vi "Build.vi"() -> ()   [LabVIEW 2010]
doc: "This VI is an example of a VI that can build a VIPM Package when the Build button is pushed or when called from the command line."
uses:
  <vilib>/Utility/error.llb/DialogType.ctl
  Types/Command Line Args.ctl
  Types/Task Info.ctl
  Types/Job Type.ctl
  <userlib>/_OpenG.lib/file/file.llb/File Exists - Scalar__ogtk.vi
  <userlib>/_OpenG.lib/file/file.llb/Valid Path - Traditional__ogtk.vi
panel:
  out "Tests Pass":bool
  out "Unit Test Results":string
  in  "Autobuild Spec":path
  in  "button_build":bool
  out "Progress status":string
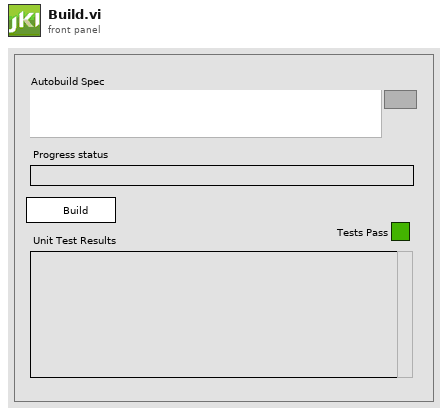
[diagram p1: front panel]
types:
  T1 = enum16{"open", "replace", "create", "open or create", "replace or create", "replace or create with confirmation"}
  T2 = enum32{"invalid app kind", "Development System", "Run Time System", "Student Edition", "Embedded LabVIEW", "Evaluation", "Custom"}
  T3 = typedef "Command Line Args.ctl" = cluster{"BuildNumber":u32, "Error":path, "Running":path, "Workspace":path, "Job":string, "MClog":path, "BuildLog":path, "Copy Built":bool, "SourceVer":string, "MaxBuildVer":string}
  T4 = enum8{"Enabled", "Disabled", "Disabled and Grayed Out"}
  T5 = enum32{"Invalid", "Standard", "Closed", "Hidden", "Minimized", "Maximized"}
  T6 = typedef "Task Info.ctl" = cluster{"Build Spec":string, "Path":path, "Target":string, "Type":T7, "Raw Command":string}
  T7 = typedef "Job Type.ctl" = enum16{"MC", "NOP", "VI", "Build", "VIP", "VIPB", "VIA"}
  T8 = cluster{"Core":cluster{"Current VI Reference":refnum<vi>, "Close Panel on Exit?":bool}, "Build":cluster{"Unit Test":path, "Builds":T6[], "Retain Build":bool}, "Building":bool, "RunningAsCmdLine":bool, "CmdLineArgs":T3, "Autobuild Spec":path, "MCSpec":path}
  T9 = typedef "DialogType.ctl" = u16
  T10 = cluster{"Unit Test":path, "Builds":T6[], "Retain Build":bool}
  T11 = cluster{"Current VI Reference":refnum<vi>, "Close Panel on Exit?":bool}
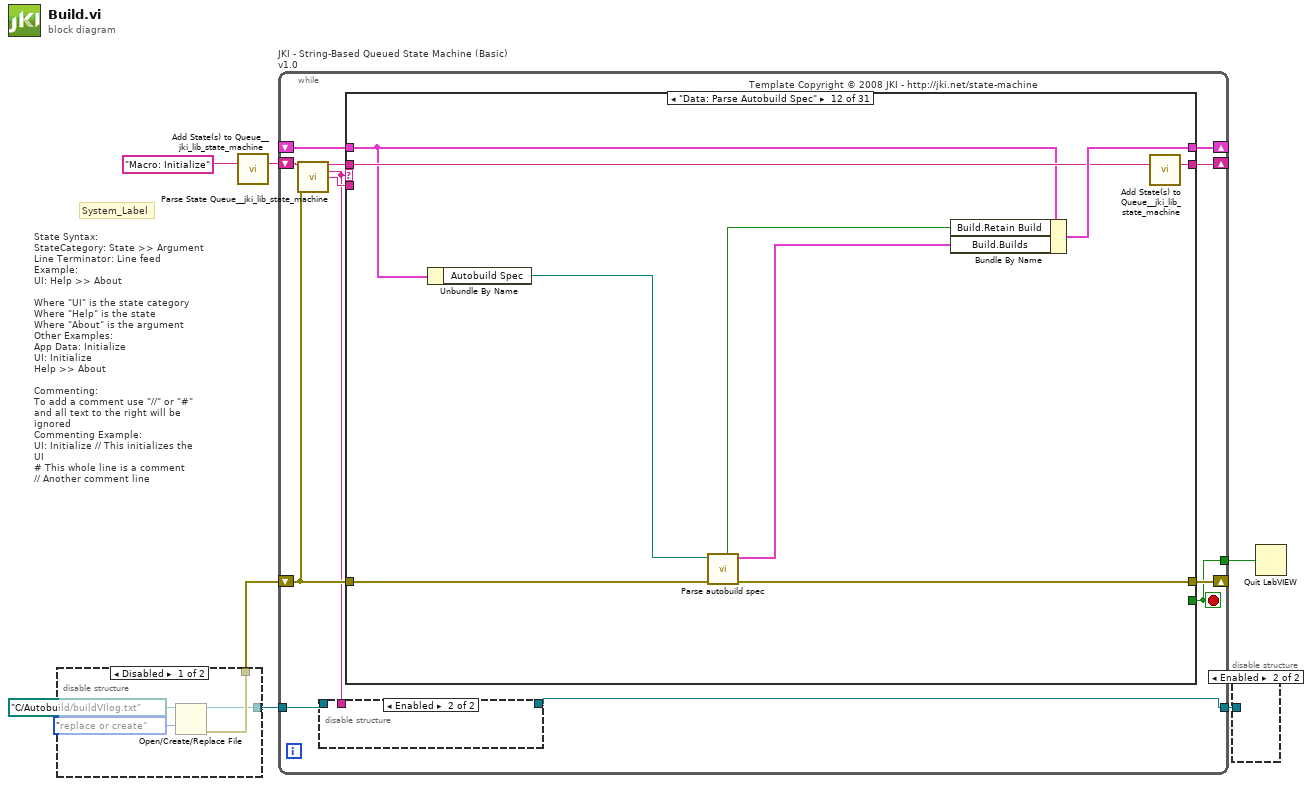
[diagram p0: block diagram]
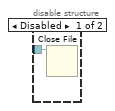
[diagram p2: hidden frame]
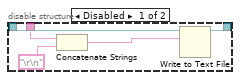
[diagram p4: hidden frame]
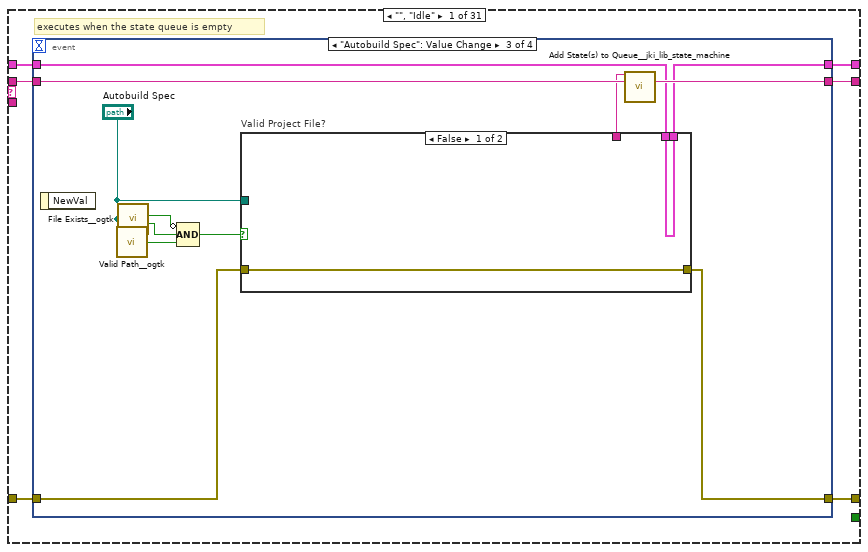
[diagram p5: hidden frame]
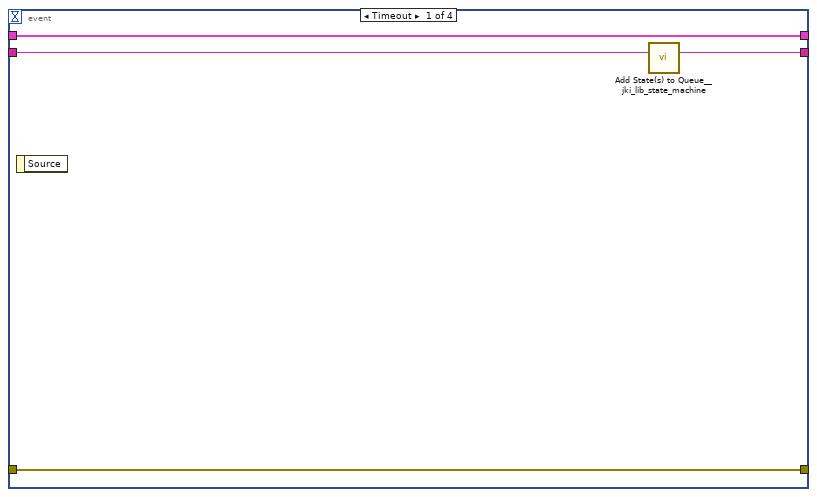
[diagram p6: hidden frame]
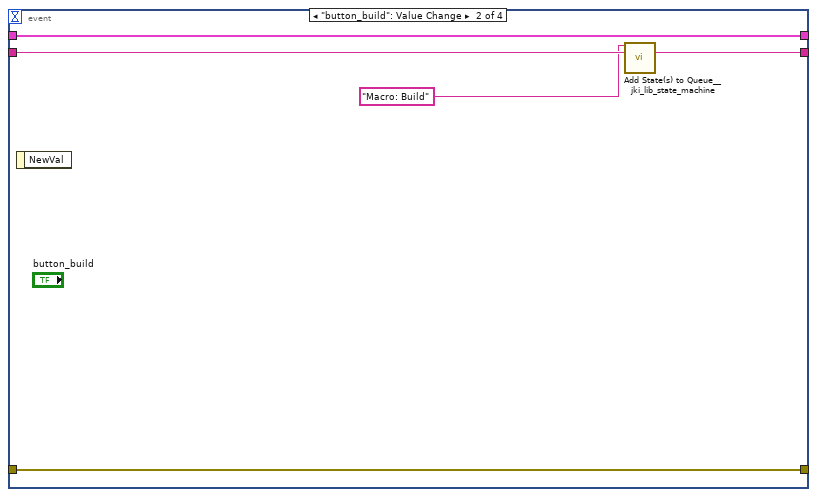
[diagram p7: hidden frame]
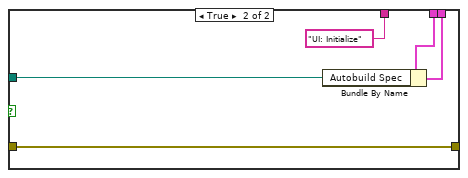
[diagram p8: hidden frame]
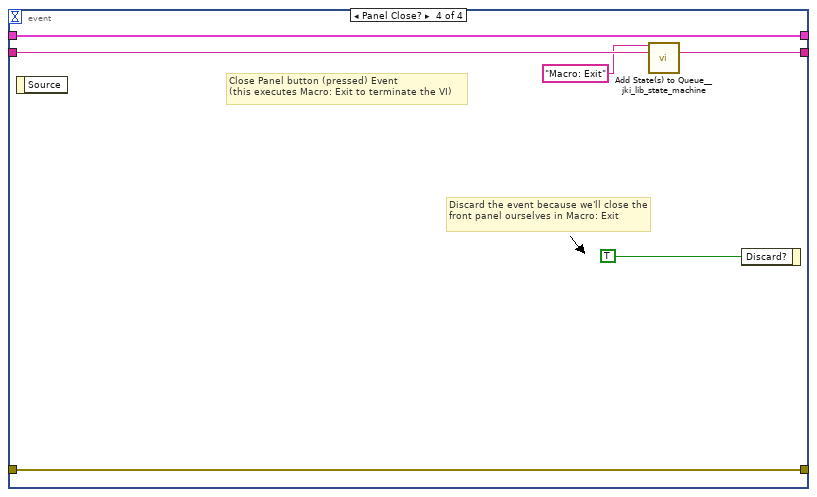
[diagram p9: hidden frame]
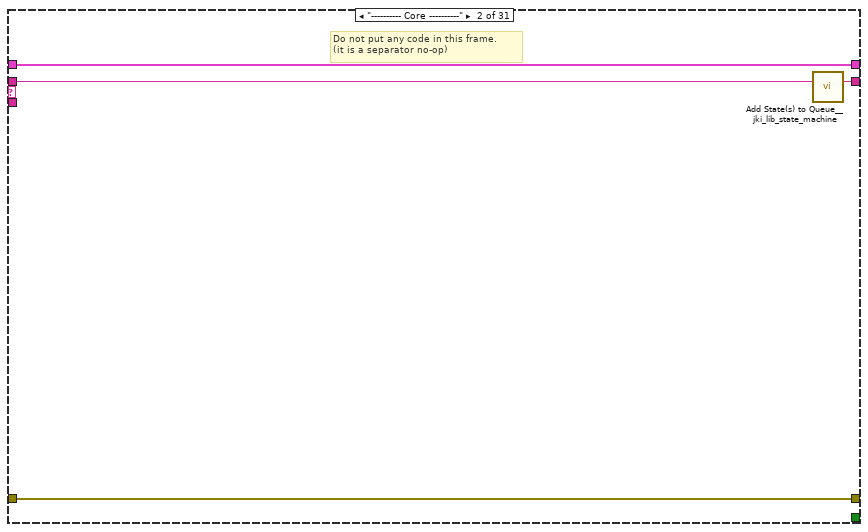
[diagram p10: hidden frame]
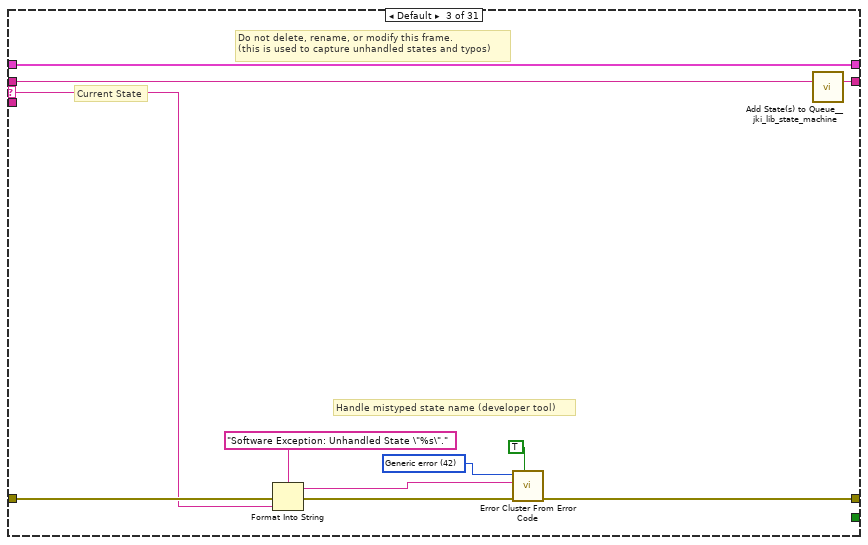
[diagram p11: hidden frame]
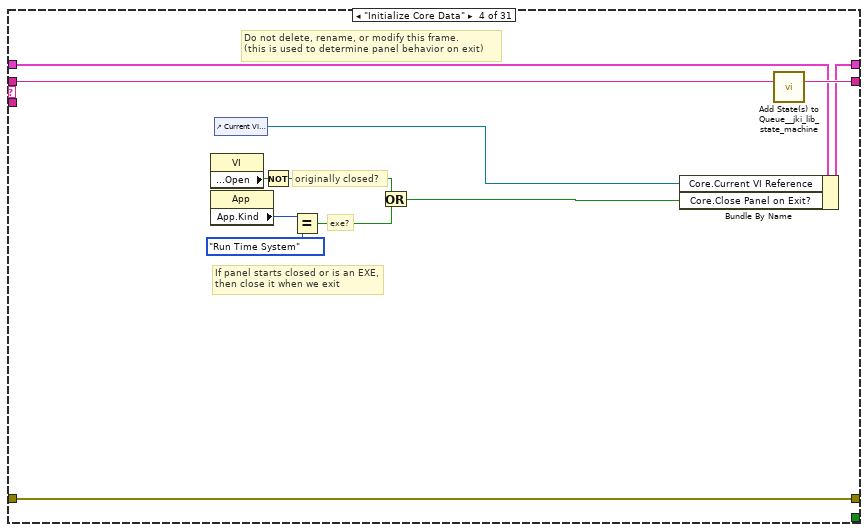
[diagram p12: hidden frame]
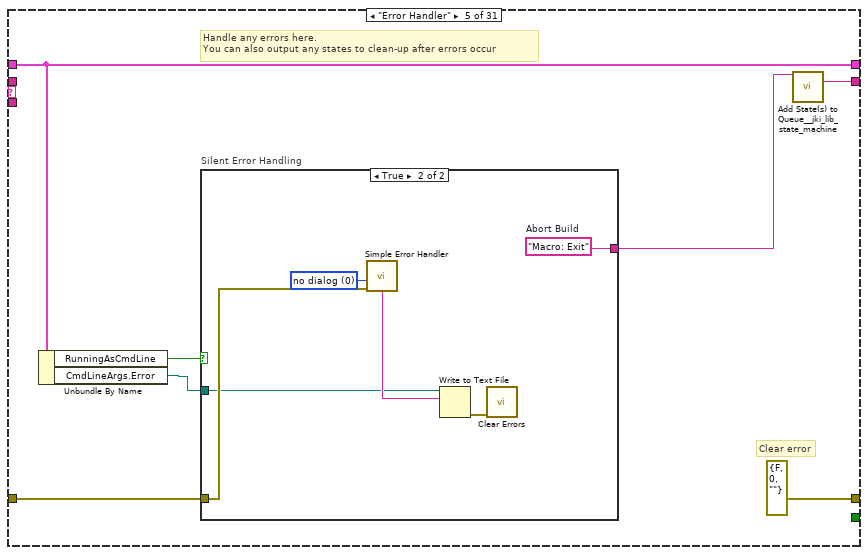
[diagram p13: hidden frame]
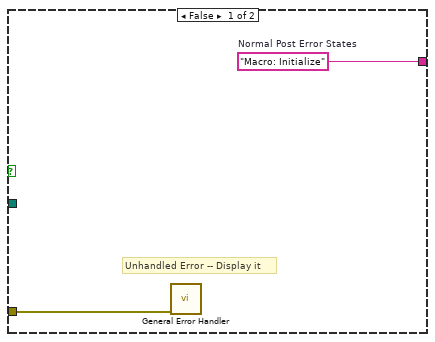
[diagram p14: hidden frame]
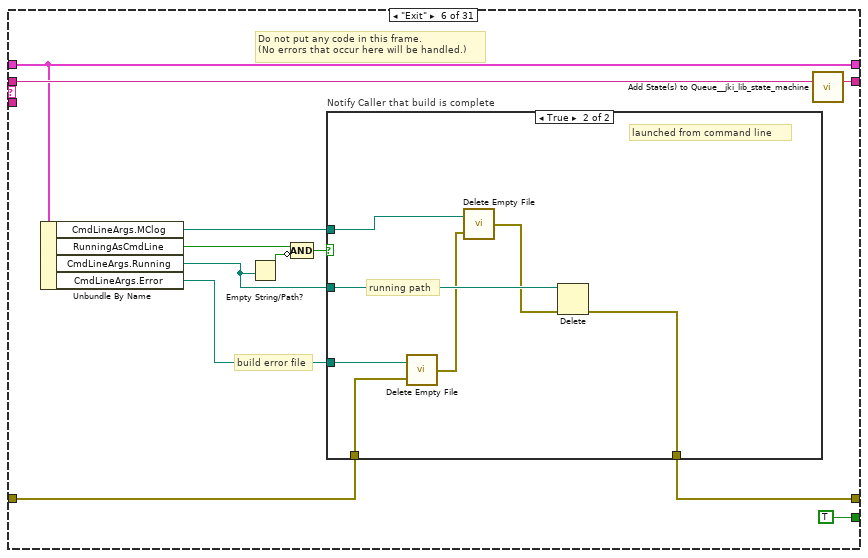
[diagram p15: hidden frame]
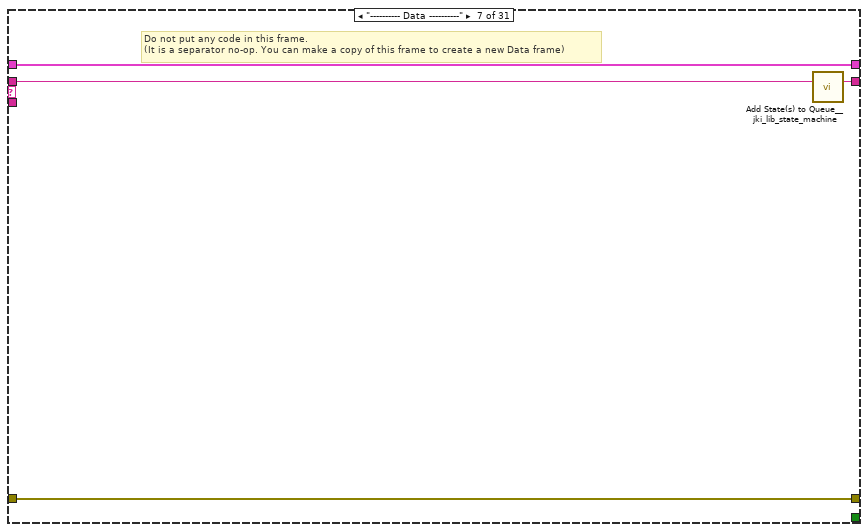
[diagram p17: hidden frame]
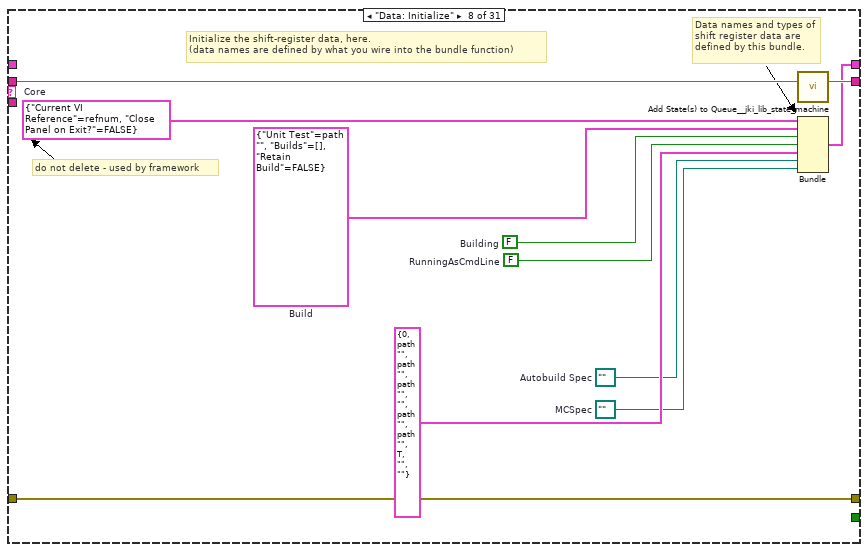
[diagram p18: hidden frame]
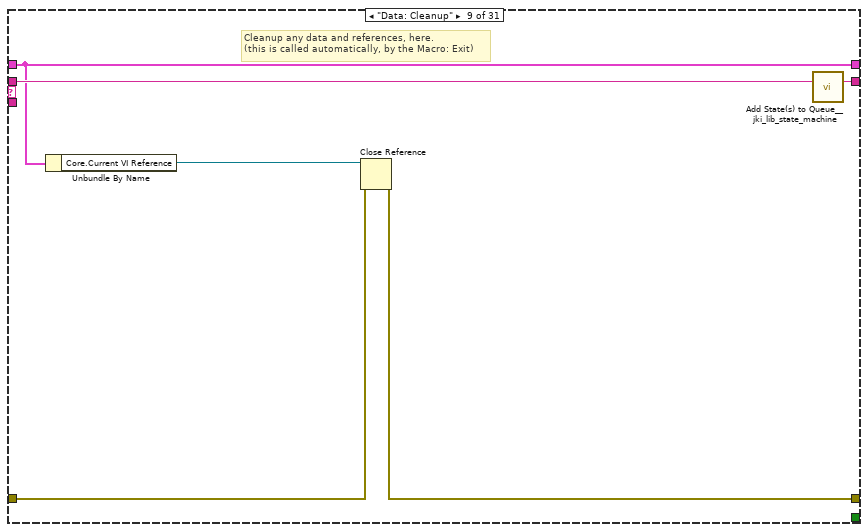
[diagram p19: hidden frame]
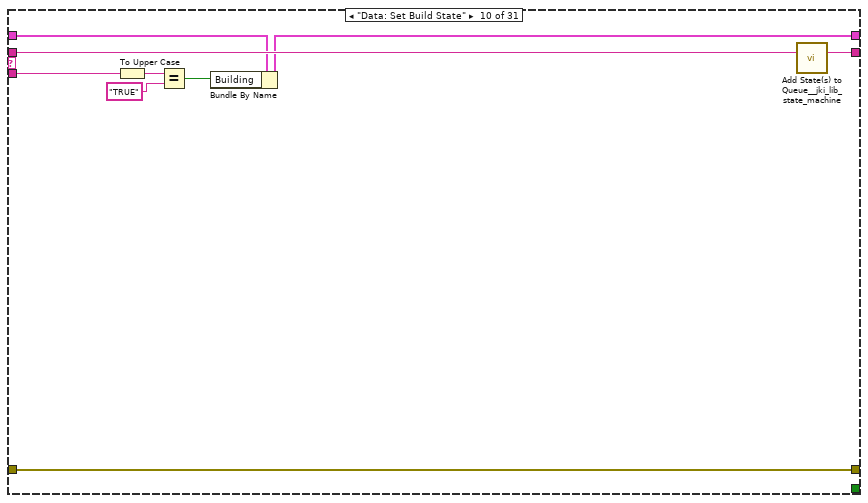
[diagram p20: hidden frame]
diagram:
  # "State Syntax:\nStateCategory: State >> Argument\nLine Terminator: Line feed\nExample:\nUI: Help >> About\n\nWhere \"UI\" is the state category\nWhere \"Help\" is the state\nWhere \"About\" is the argument\nOther Examples:\nApp Data: Initialize\nUI: Initialize\nHelp >> About\n\nCommenting:\nTo add a comment use \"//\" or \"#\" and all text to the right will be ignored\nCommenting Example:\nUI: Initialize // This initializes the UI\n# This whole line is a comment\n// Another comment line"
  # "System_Label"
  n1 = disable-structure shown="Disabled" {
    disable-tunnel: [w10 _] -> w4
    disable-tunnel: [w8 _] -> w3
    frame Disabled {
      n2 = Open/Create/Replace File(file path (use dialog)=path "C:/Autobuild/buildVIlog.txt", operation (0:open)=T1."replace or create") -> (refnum out=w8:refnum<file>, error out=w10:errorcluster)  [unwired: 4 in, 1 out]
    }
    frame Enabled {
    }
  }
  n3 = call <vilib>:"Add State(s) to Queue__jki_lib_state_machine.vi"("State(s) in (\"\")"="Macro: Initialize") -> ("States Out"=w5:string)  [unwired: 14 in]
  n4 = while "JKI - String-Based Queued State Machine (Basic) v1.0" {
    shift-right: [w17] -> _
    shift-left: _ -> [w16]
    shift-right: [w19] -> _
    shift-left: w4 -> [w15]
    shift-right: [w18] -> _
    shift-left: w5 -> [w20]
    tunnel: w3 -> [w14]
    tunnel: [w11] -> w2
    tunnel: [w12] -> w1
    stop <- w12 stop-if-true
    # "Template Copyright © 2008 JKI - http://jki.net/state-machine"
    n5 = call <vilib>:"Parse State Queue__jki_lib_state_machine.vi"("State Queue"=w20, "Error In (no error)"=w15) -> ("Remaining States"=w22:string, "Current State"=w13:string, "Arguments"=w21:string)  [unwired: 11 in]
    n6 = disable-structure shown="Enabled" {
      disable-tunnel: w14 -> [w27 _]
      disable-tunnel: w13 -> [w26 _]
      disable-tunnel: [w23 _] -> w11
      frame Disabled {
        n7 = Concatenate Strings(w26, "\r\n") -> (w25:string)
        n8 = Write to Text File(file (use dialog)=w27, text=w25) -> (refnum out=w23:refnum<file>)  [unwired: 2 in, 2 out]
      }
      frame Enabled {
      }
    }
    n9 = case shown="\"Data: Parse Autobuild Spec\"" w13 {
      selector: w13 -> [_ _ w72 _ _ _ _ _ _ _ _ _ _ _ _ _ _ _ _ _ _ _ _ _ _ _ _ _ _ _ _]
      tunnel: w22 -> [w33 w71 w76 w94 _ w121 w133 w144 w150 w159 w198 w207 w213 w222 w227 w232 w240 w246 w257 w283 w288 w293 w298 w303 w313 w317 w336 w359 w382 w406 w421]
      tunnel: w21 -> [_ _ _ _ _ _ _ _ _ w153 _ _ _ _ _ w228 _ w241 w251 _ _ _ _ _ _ _ _ _ _ _ _]
      tunnel: w16 -> [w31 w68 w74 w85 w99 w111 w130 _ w145 w157 w196 w206 w210 w220 w225 w230 w238 w244 w253 w280 w285 w290 w296 w300 w310 w314 w338 w357 w380 w404 w419]
      tunnel: [w30 w69 w78 w91 errorcluster {"status"=FALSE, "code"=0, "source"=""} ("error out") w110 w131 w140 w146 w156 w192 w202 w211 w216 w224 w229 w237 w242 w254 w281 w286 w291 w295 w301 w311 w315 w324 w354 w372 w401 w413] -> w19
      tunnel: w15 -> [w29 w69 w77 w91 w97 w118 w131 w140 w147 w156 w192 w205 w211 w219 w224 w229 w237 w243 w255 w281 w286 w291 w295 w301 w311 w315 w329 w356 w379 w403 w416]
      tunnel: [w32 w70 w75 w93 w101 w120 w132 w143 w149 w158 w197 w209 w212 w221 w226 w231 w239 w245 w256 w282 w287 w292 w297 w302 w312 w316 w339 w358 w381 w405 w420] -> w18
      tunnel: [_ _ _ _ _ TRUE _ _ _ _ _ _ _ _ _ _ _ _ _ _ _ _ _ _ _ _ _ _ _ _ _] -> w12
      tunnel: [w28 w68 w74 w92 w99 w111 w130 w142 w145 w155 w195 w208 w210 w220 w225 w230 w238 w244 w253 w280 w285 w290 w296 w300 w310 w314 w338 w357 w380 w404 w419] -> w17
      frame "", "Idle" {
        # "executes when the state queue is empty"
        n10 = event shown="[2] \"Autobuild Spec\": Value Change" {
          selector: _ -> [_ _ _ _]
          dyn-events: _ -> [_ _ _ _]
          timeout: _ -> [_ _ _ _]
          tunnel: w33 -> [w37 w42 w54 w67]
          tunnel: [w36 w41 w53 w66] -> w32
          tunnel: w31 -> [w34 w38 w48 w64]
          tunnel: [w35 w39 w44 w65] -> w30
          tunnel: w29 -> [w35 w39 w45 w65]
          tunnel: [w34 w38 w47 w64] -> w28
          event Timeout {
            n11 = event-data() -> ()  [unwired: 1 in, 1 out]
            n12 = call <vilib>:"Add State(s) to Queue__jki_lib_state_machine.vi"("State(s) in (\"\")"=w37) -> ("States Out"=w36:string)  [unwired: 14 in]
          }
          event "button_build": Value Change {
            n13 = event-data() -> ()  [unwired: 1 in, 1 out]
            n14 = call <vilib>:"Add State(s) to Queue__jki_lib_state_machine.vi"("State(s) in Front (\"\")"="Macro: Build", "State(s) in (\"\")"=w42) -> ("States Out"=w41:string)  [unwired: 13 in]
          }
          event "Autobuild Spec": Value Change {
            n15 = event-data() -> ()  [unwired: 1 in, 1 out]
            n16 = call-poly <userlib>:"Valid Path__ogtk.vi"("path"="Autobuild Spec") -> ("valid"=w52:bool)
            n17 = call-poly <userlib>:"File Exists__ogtk.vi"("file path"="Autobuild Spec") -> ("is directory"=w50:bool, "exists"=w51:bool)  [unwired: 6 in]
            n18 = Compound Arithmetic op=AND(invert w50, w51, w52) -> (w49:bool)
            n19 = case "Valid Project File?" shown="False" w49 {
              tunnel: w45 -> [w56 w57]
              tunnel: "Autobuild Spec" -> [_ w59]
              tunnel: w48 -> [w55 w61]
              tunnel: [w55 w60] -> w47
              tunnel: [_ "UI: Initialize"] -> w46
              tunnel: [w56 w57] -> w44
              frame False {
              }
              frame True {
                n20 = Bundle By Name(cluster=w61, "Autobuild Spec"=w59) -> (w60:T8)
              }
            }
            n21 = call <vilib>:"Add State(s) to Queue__jki_lib_state_machine.vi"("State(s) in Front (\"\")"=w46, "State(s) in (\"\")"=w54) -> ("States Out"=w53:string)  [unwired: 13 in]
          }
          event Panel Close? {
            # "Discard the event because we'll close the front panel ourselves in Macro: Exit"
            # "Close Panel button (pressed) Event\n(this executes Macro: Exit to terminate the VI)"
            n22 = event-data() -> ()  [unwired: 1 in, 1 out]
            n23 = call <vilib>:"Add State(s) to Queue__jki_lib_state_machine.vi"("State(s) in Front (\"\")"="Macro: Exit", "State(s) in (\"\")"=w67) -> ("States Out"=w66:string)  [unwired: 13 in]
            n24 = event-data("Discard?"=TRUE) -> ()  [unwired: 1 in, 1 out]
          }
        }
      }
      frame "---------- Core ----------" {
        # "Do not put any code in this frame.\n(it is a separator no-op)"
        n25 = call <vilib>:"Add State(s) to Queue__jki_lib_state_machine.vi"("State(s) in (\"\")"=w71) -> ("States Out"=w70:string)  [unwired: 14 in]
      }
      frame Default {
        w81 = 42 items=["No error", "Argument error", "Memory is full", "Out of zone", "End of file", "File already open", "Generic file I/O error", "File not found", "File permission error", "Disk is full", "Duplicate path", "Too many files open", "System feature not enabled", "Resource file not found", "Cannot add resource", "Resource not found", "Image not found", "Image memory error", "Pen does not exist", "Config type invalid", "Config token not found", "Config parse error", "Config memory error", "Bad external code format", "Bad external code offset", "External code not present", "Null window", "Destroy window error", "Null menu", "Print aborted", "Bad print record", "Print driver error", "Windows error during printing", "Memory error during printing", "Print dialog error", "Generic print error", "Invalid device refnum", "Device not found", "Device parameter error", "Device unit error", "Cannot open device", "Device call aborted", "Generic error", "Cancelled by user", "Object ID too low", "Object ID too high", "Object not in heap", "Unknown heap", "Unknown object (invalid DefProc)", "Unknown object (DefProc not in table)", "Message out of range", "Invalid (null) method", "Unknown message", "Manager call not supported", "Bad address", "Network operation in progress", "Network operation timed out", "Connection is busy", "Network attribute not supported", "Network error", "Address in use", "System out of memory", "Connection aborted", "Connection refused", "Not connected", "Already connected", "Connection closed", "Initialization error (interapplication manager)", "Bad occurrence", "Wait on unbound occurrence handler", "Occurrence queue overflow", "Datalog type conflict", "Unused", "Unrecognized type (interapplication manager)", "Memory corrupt", "Failed to make temporary DLL", "Old CIN version", "Drag socket not found", "Failed to load drop-object", "Failed to register OLE object", "Failed to release OLE object", "Format specifier type mismatch", "Unknown format specifier", "Too few format specifiers", "Too many format specifiers", "Scan failed", "Newer CIN version", "Error converting to variant", "Runtime menu error", "Password tampered", "Variant attribute not found", "Incompatible variant data type", "Event data is not available", "Event Store is not present", "Occurrence is not found", "Event Queue is not created", "Event info is not available", "Refnum passed is NULL", "Error retrieving Class GUID", "Error retrieving CoClass GUID", "Error retrieving TypeLib GUID.", "Bad built application magic bytes.", "Specific driver is different from the specific driver associated with the Logical Name.", "There is no session opened to the class driver.", "Max Error", "MAX - Error with config objects", "MAX - Error loading configuration", "MAX - Group not supported"]
        # "Current State"
        # "Do not delete, rename, or modify this frame.\n(this is used to capture unhandled states and typos)"
        # "Handle mistyped state name (developer tool)"
        n26 = Format Into String(format string="Software Exception: Unhandled State \"%s\"." ("message"), error in=w77, w72) -> (resulting string=w80:string, error out=w79:errorcluster)  [unwired: 1 in]
        n27 = call <vilib>:"Error Cluster From Error Code.vi"("show call chain? (False)"=TRUE, "error in (no error)"=w79, "error message (\"\")"=w80, "error code (0)"=w81) -> ("error out"=w78:errorcluster)  [unwired: 5 in]
        n28 = call <vilib>:"Add State(s) to Queue__jki_lib_state_machine.vi"("State(s) in (\"\")"=w76) -> ("States Out"=w75:string)  [unwired: 14 in]
      }
      frame "Initialize Core Data" {
        # "Do not delete, rename, or modify this frame.\n(this is used to determine panel behavior on exit)"
        # "originally closed?"
        # "exe?"
        # "If panel starts closed or is an EXE, then close it when we exit"
        n29 = property class="VI"() -> ("Front Panel.Open"=w90:bool)  [unwired: 2 in, 2 out]
        n30 = property class="App"() -> ("App.Kind"=w89:T2)  [unwired: 2 in, 2 out]
        n31 = control-ref of="Current VI Reference"() -> (w83:refnum<vi>)
        n32 = Not(x=w90) -> (.not. x?=w87:bool)
        n33 = Equal?(x=w89, y=T2."Run Time System" ("Application:Kind")) -> (x = y?=w86:bool)
        n34 = Or(x=w87, y=w86) -> (x .or. y?=w84:bool)
        n35 = Bundle By Name(cluster=w85, "Core.Current VI Reference"=w83, "Core.Close Panel on Exit?"=w84) -> (w92:T8)
        n36 = call <vilib>:"Add State(s) to Queue__jki_lib_state_machine.vi"("State(s) in (\"\")"=w94) -> ("States Out"=w93:string)  [unwired: 14 in]
      }
      frame "Error Handler" {
        # "Handle any errors here.\nYou can also output any states to clean-up after errors occur"
        # "Clear error"
        n37 = Unbundle By Name(w99) -> ("RunningAsCmdLine"=w98:bool, "CmdLineArgs.Error"=w95:path)
        n38 = case "Silent Error Handling" shown="True" w98 {
          tunnel: w97 -> [w103 w106]
          tunnel: [w102 w108] -> w96
          tunnel: w95 -> [_ w105]
          frame False {
            w102 = "Macro: Initialize"  # Normal Post Error States
            # "Unhandled Error -- Display it"
            n39 = call <vilib>:"General Error Handler.vi"("error in (no error)"=w103) -> ()  [unwired: 10 in, 5 out]
          }
          frame True {
            w104 = T9 0 items=["no dialog", "OK message", "continue or stop message", "OK message + warnings", "continue/stop + warnings"] ("type of dialog (OK msg:1)")
            w108 = "Macro: Exit"  # Abort Build
            n40 = call <vilib>:"Simple Error Handler.vi"("type of dialog (OK msg:1)"=w104, "error in (no error)"=w106) -> ("message"=w109:string)  [unwired: 3 in, 4 out]
            n41 = Write to Text File(file (use dialog)=w105, text=w109) -> (error out=w107:errorcluster)  [unwired: 2 in, 2 out]
            n42 = call <vilib>:"Clear Errors.vi"("error in (no error)"=w107) -> ()  [unwired: 6 in, 1 out]
          }
        }
        n43 = call <vilib>:"Add State(s) to Queue__jki_lib_state_machine.vi"("State(s) in Front (\"\")"=w96) -> ("States Out"=w101:string)  [unwired: 14 in]
      }
      frame "Exit" {
        # "build error file"
        # "Do not put any code in this frame.\n(No errors that occur here will be handled.)"
        n44 = Unbundle By Name(w111) -> ("CmdLineArgs.MClog"=w112:path, "RunningAsCmdLine"=w117:bool, "CmdLineArgs.Running"=w114:path, "CmdLineArgs.Error"=w113:path)
        n45 = Empty String/Path?(string/path=w114) -> (empty?=w116:bool)
        n46 = Compound Arithmetic op=AND(w117, invert w116) -> (w115:bool)
        n47 = case "Notify Caller that build is complete" shown="True" w115 {
          tunnel: w114 -> [_ w126]
          tunnel: w118 -> [w122 w128]
          tunnel: [w122 w129] -> w110
          tunnel: w113 -> [_ w127]
          tunnel: w112 -> [_ w123]
          frame False {
          }
          frame True {
            # "running path"
            # "launched from command line"
            n48 = call "Delete Empty File.vi"("error in"=w128, "Path"=w127) -> ("error out"=w125:errorcluster)
            n49 = call "Delete Empty File.vi"("error in"=w125, "Path"=w123) -> ("error out"=w124:errorcluster)
            n50 = Delete(path (use dialog)=w126, error in=w124) -> (error out=w129:errorcluster)  [unwired: 3 in, 2 out]
          }
        }
        n51 = call <vilib>:"Add State(s) to Queue__jki_lib_state_machine.vi"("State(s) in (\"\")"=w121) -> ("States Out"=w120:string)  [unwired: 14 in]
      }
      frame "---------- Data ----------" {
        # "Do not put any code in this frame.\n(It is a separator no-op. You can make a copy of this frame to create a new Data frame)"
        n52 = call <vilib>:"Add State(s) to Queue__jki_lib_state_machine.vi"("State(s) in (\"\")"=w133) -> ("States Out"=w132:string)  [unwired: 14 in]
      }
      frame "Data: Initialize" {
        w134 = path ""  # MCSpec
        w135 = path ""  # Autobuild Spec
        w138 = FALSE  # RunningAsCmdLine
        w136 = T10 {"Unit Test"=path "", "Builds"=[], "Retain Build"=FALSE}  # Build
        w139 = FALSE  # Building
        w141 = T11 {"Current VI Reference"=refnum, "Close Panel on Exit?"=FALSE}  # Core
        # "do not delete - used by framework"
        # "Data names and types of shift register data are defined by this bundle."
        # "Initialize the shift-register data, here.\n(data names are defined by what you wire into the bundle function)"
        n53 = call <vilib>:"Add State(s) to Queue__jki_lib_state_machine.vi"("State(s) in (\"\")"=w144) -> ("States Out"=w143:string)  [unwired: 14 in]
        n54 = Bundle("Core"=w141, "Build"=w136, "Building"=w139, "RunningAsCmdLine"=w138, "CmdLineArgs"=T3 {"BuildNumber"=0, "Error"=path "", "Running"=path "", "Workspace"=path "", "Job"="", "MClog"=path "", "BuildLog"=path "", "Copy Built"=TRUE, "SourceVer"="", "MaxBuildVer"=""}, "Autobuild Spec"=w135, "MCSpec"=w134) -> (w142:T8)  [unwired: 1 in]
      }
      frame "Data: Cleanup" {
        # "Cleanup any data and references, here.\n(this is called automatically, by the Macro: Exit)"
        n55 = Unbundle By Name(w145) -> ("Core.Current VI Reference"=w148:refnum<vi>)
        n56 = Close Reference(reference=w148, error in (no error)=w147) -> (error out=w146:errorcluster)
        n57 = call <vilib>:"Add State(s) to Queue__jki_lib_state_machine.vi"("State(s) in (\"\")"=w150) -> ("States Out"=w149:string)  [unwired: 14 in]
      }
      frame "Data: Set Build State" {
        n58 = To Upper Case(1:w153) -> (0:w154:string)
        n59 = Equal?(x=w154, y="TRUE") -> (x = y?=w151:bool)
        n60 = Bundle By Name(cluster=w157, "Building"=w151) -> (w155:T8)
        n61 = call <vilib>:"Add State(s) to Queue__jki_lib_state_machine.vi"("State(s) in (\"\")"=w159) -> ("States Out"=w158:string)  [unwired: 14 in]
      }
      frame "Data: Command Line Handler" {
        # "next BuildNumber"
        n62 = property class="App"() -> ("App.Args"=w160:string[])  [unwired: 2 in, 2 out]
        n63 = Index Array(array=w160, index #1=1, index #9=10 ("index"), index #10=11 ("index"), index #11=9 ("index")) -> (element #1=w186:string, element #2=w184:string, element #3=w181:string, element #4=w179:string, element #5=w178:string, element #6=w177:string, element #7=w176:string, element #8=w174:string, element #9=w170:string, element #10=w166:string, element #11=w164:string)  [unwired: 7 in]
        n64 = case shown="Default" w170 {
          tunnel: [TRUE FALSE] -> w169
          frame Default {
          }
          frame "0", "f", "false", "n", "no" {
          }
        }
        n65 = String To Path(string=w184) -> (path=w182:path)
        n66 = String To Path(string=w181) -> (path=w180:path)
        n67 = String To Path(string=w179) -> (path=w171:path)
        n68 = String To Path(string=w176) -> (path=w175:path)
        n69 = String To Path(string=w174) -> (path=w173:path)
        n70 = Array Size(array=w160) -> (size(s)=w191:i32)
        n71 = Greater?(x=w191, y=1) -> (0:w189:bool)
        n72 = Decimal String To Number(string=w186, default (0L)=u32 0 ("Package Version.build")) -> (number=w183:u32)  [unwired: 1 in, 1 out]
        n73 = Concatenate Strings("Autobuild" ("name or relative path"), w166, ".csv" ("name or relative path")) -> (w165:string)
        n74 = Build Path(base path=w171, name or relative path=w165) -> (appended path=w172:path)
        n75 = Bundle By Name(cluster=w196, "RunningAsCmdLine"=w189, "CmdLineArgs.BuildNumber"=w183, "CmdLineArgs.Error"=w182, "CmdLineArgs.Running"=w180, "CmdLineArgs.Workspace"=w171, "CmdLineArgs.Job"=w178, "Autobuild Spec"=w172, "CmdLineArgs.SourceVer"=w177, "CmdLineArgs.MClog"=w175, "CmdLineArgs.BuildLog"=w173, "CmdLineArgs.Copy Built"=w169, "CmdLineArgs.MaxBuildVer"=w164) -> (w195:T8)
        n76 = Select(t="Macro: Build\nMacro: Exit", s=w189, f="") -> (s? t:f=w193:string)
        n77 = call <vilib>:"Add State(s) to Queue__jki_lib_state_machine.vi"("State(s) in Front (\"\")"=w193, "State(s) in (\"\")"=w198) -> ("States Out"=w197:string)  [unwired: 13 in]
      }
      frame "Data: Parse Autobuild Spec" {
        n78 = Unbundle By Name(w206) -> ("Autobuild Spec"=w204:path)
        n79 = call "Parse autobuild spec.vi"("error in"=w205, "Autobuild spec"=w204) -> ("error out"=w202:errorcluster, "Tasks"=w203:T6[], "Retain Build"=w201:bool)  [unwired: 7 in]
        n80 = Bundle By Name(cluster=w206, "Build.Retain Build"=w201, "Build.Builds"=w203) -> (w208:T8)
        n81 = call <vilib>:"Add State(s) to Queue__jki_lib_state_machine.vi"("State(s) in (\"\")"=w207) -> ("States Out"=w209:string)  [unwired: 14 in]
      }
      frame "---------- UI ----------" {
        # "Do not put any code in this frame.\n(It is a separator no-op. You can make a copy of this frame to create a new UI frame)"
        n82 = call <vilib>:"Add State(s) to Queue__jki_lib_state_machine.vi"("State(s) in (\"\")"=w213) -> ("States Out"=w212:string)  [unwired: 14 in]
      }
      frame "UI: Initialize" {
        # "Initialize the User Interface, here.\n(this is called automatically, by the Macro: Init)"
        n83 = Unbundle By Name(w220) -> ("Autobuild Spec"=w215:path)
        n84 = local write "Autobuild Spec"(w215) -> ()
        n85 = call <userlib>:"Fit VI window to Largest Dec__ogtk.vi"("error in (no error)"=w219, "border spacing (2 px)"=-1) -> ("error out"=w216:errorcluster)  [unwired: 4 in, 1 out]
        n86 = local write "Tests Pass"(FALSE ("Unit Tests Pass")) -> ()
        n87 = local write "Unit Test Results"("") -> ()
        n88 = call <vilib>:"Add State(s) to Queue__jki_lib_state_machine.vi"("State(s) in (\"\")"=w222) -> ("States Out"=w221:string)  [unwired: 14 in]
      }
      frame "UI: Reset Progress Status" {
        n89 = call <vilib>:"Add State(s) to Queue__jki_lib_state_machine.vi"("State(s) in Front (\"\")"="UI: Update Progress Status >> Idle" ("State(s) in Front (\"\")"), "State(s) in (\"\")"=w227) -> ("States Out"=w226:string)  [unwired: 13 in]
      }
      frame "UI: Update Progress Status" {
        n90 = call <vilib>:"Add State(s) to Queue__jki_lib_state_machine.vi"("State(s) in (\"\")"=w232) -> ("States Out"=w231:string)  [unwired: 14 in]
        "Progress status" <- w228
      }
      frame "UI: Update Interlock" {
        n91 = Unbundle By Name(w238) -> ("Building"=w234:bool)
        n92 = Select(t=T4."Disabled and Grayed Out" ("Disabled"), s=w234, f=T4."Enabled" ("Disabled")) -> (s? t:f=w233:T4)
        n93 = property on="button_build" class="Bool"("DisabledEnum"=w233) -> ()  [unwired: 2 in, 2 out]
        n94 = property on="Autobuild Spec" class="Path"("DisabledEnum"=w233) -> ()  [unwired: 2 in, 2 out]
        n95 = call <vilib>:"Add State(s) to Queue__jki_lib_state_machine.vi"("State(s) in (\"\")"=w240) -> ("States Out"=w239:string)  [unwired: 14 in]
      }
      frame "UI: Cursor Set" {
        # "Argument"
        # "Set and Unset Cursor Busy.\n(Usage: \"UI: Cursor Set >> Busy|Idle\")"
        n96 = case shown="\"Idle\", Default" w241 {
          tunnel: w243 -> [w248 w250]
          tunnel: [w247 w249] -> w242
          frame "Idle", Default {
            n97 = call <vilib>:"Unset Busy.vi"("error in (no error)"=w248) -> ("error out"=w247:errorcluster)  [unwired: 10 in]
          }
          frame "Busy" {
            n98 = call <vilib>:"Set Busy.vi"("error in (no error)"=w250) -> ("error out"=w249:errorcluster)  [unwired: 9 in, 1 out]
          }
        }
        n99 = call <vilib>:"Add State(s) to Queue__jki_lib_state_machine.vi"("State(s) in (\"\")"=w246) -> ("States Out"=w245:string)  [unwired: 14 in]
      }
      frame "UI: Front Panel State" {
        # "Argument"
        # "Set Front Panel Open or Closed\n(Usage: \"UI: Front Panel State >> Open|Close\")"
        n100 = Unbundle By Name(w253) -> ("Core.Current VI Reference"=w252:refnum<vi>)
        n101 = case shown="\"Open\", Default" w251 {
          tunnel: w255 -> [w261 w274]
          tunnel: [w263 w275] -> w254
          tunnel: w252 -> [w262 w272]
          frame "Open", Default {
            n102 = property class="VI"(reference=w262, error in=w261) -> (reference out=w259:refnum<vi>, error out=w260:errorcluster, "Front Panel.Open"=w258:bool)
            n103 = case shown="False" w258 {
              tunnel: [w266 w269] -> w263
              tunnel: w260 -> [w265 w269]
              tunnel: w259 -> [w264 _]
              frame False {
                n104 = invoke class="VI" method="FP.Open"(reference=w264, error in=w265, "Activate"=TRUE, "State"=T5."Standard") -> (error out=w266:errorcluster)  [unwired: 1 in, 4 out]
              }
              frame True {
              }
            }
          }
          frame "Close" {
            n105 = property class="VI"(reference=w272, error in=w274) -> (reference out=w271:refnum<vi>, error out=w273:errorcluster, "Front Panel.Open"=w270:bool)
            n106 = case shown="True" w270 {
              tunnel: [w276 w279] -> w275
              tunnel: w273 -> [w276 w278]
              tunnel: w271 -> [_ w277]
              frame False {
              }
              frame True {
                n107 = invoke class="VI" method="FP.Close"(reference=w277, error in=w278) -> (error out=w279:errorcluster)  [unwired: 1 in, 2 out]
              }
            }
          }
        }
        n108 = call <vilib>:"Add State(s) to Queue__jki_lib_state_machine.vi"("State(s) in (\"\")"=w257) -> ("States Out"=w256:string)  [unwired: 14 in]
      }
      frame "---------- Macro ----------" {
        # "Do not put any code in this frame.\n(It is a separator no-op. You can make a copy of this frame to create a new Macro frame)"
        n109 = call <vilib>:"Add State(s) to Queue__jki_lib_state_machine.vi"("State(s) in (\"\")"=w283) -> ("States Out"=w282:string)  [unwired: 14 in]
      }
      frame "Macro: Initialize" {
        w284 = "Data: Initialize\nInitialize Core Data\nUI: Initialize\nUI: Update Interlock\nUI: Reset Progress Status\nUI: Front Panel State >> Open\nData: Command Line Handler"  # Data: Initialize Initialize Core Data UI: Initialize UI: Update Interlock UI: Reset Progress Status UI: Front Panel State >> Open Data: Command Line Handler
        # "Initialization Macro\n(This is called once, when the VI starts)"
        n110 = call <vilib>:"Add State(s) to Queue__jki_lib_state_machine.vi"("State(s) in Front (\"\")"=w284, "State(s) in (\"\")"=w288) -> ("States Out"=w287:string)  [unwired: 13 in]
      }
      frame "Macro: Start Build" {
        # "Removed this from the template because I don't have any ability for unit tests yet"
        # "UI: Update Progress Status >> Running Unit Tests ...\nProject: Run Unit Tests"
        n111 = call <vilib>:"Add State(s) to Queue__jki_lib_state_machine.vi"("State(s) in Front (\"\")"="Data: Parse Autobuild Spec\nData: Set Build State >> True\nUI: Update Interlock", "State(s) in (\"\")"=w293) -> ("States Out"=w292:string)  [unwired: 13 in]
      }
      frame "Macro: Build" {
        n112 = call <vilib>:"Add State(s) to Queue__jki_lib_state_machine.vi"("State(s) in Front (\"\")"="Macro: Start Build\nUI: Update Progress Status >> Building ...\nProject: Copy .config\nClear Compiled Obj Cache\nProject: Build\nProject: Copy to Built\nUI: Reset Progress Status \nMacro: End Build", "State(s) in (\"\")"=w298) -> ("States Out"=w297:string)  [unwired: 13 in]
      }
      frame "Macro: End Build" {
        n113 = call <vilib>:"Add State(s) to Queue__jki_lib_state_machine.vi"("State(s) in Front (\"\")"="Data: Set Build State >> False\nUI: Update Interlock", "State(s) in (\"\")"=w303) -> ("States Out"=w302:string)  [unwired: 13 in]
      }
      frame "Macro: Exit" {
        # "Exit Macro\n(This is called once, when the VI exits)"
        n114 = Unbundle By Name(w310) -> ("Core.Close Panel on Exit?"=w309:bool)
        n115 = Select(t="UI: Front Panel State >> Close", s=w309, f="") -> (s? t:f=w306:string)
        n116 = call <vilib>:"Add State(s) to Queue__jki_lib_state_machine.vi"("State(s) in (\"\")"=w306, "State(s) at Back (\"\")"="Data: Cleanup\nExit") -> ("States Out"=w304:string)  [unwired: 13 in]
        n117 = call <vilib>:"Add State(s) to Queue__jki_lib_state_machine.vi"("State(s) in Front (\"\")"=w304, "State(s) in (\"\")"=w313) -> ("States Out"=w312:string)  [unwired: 13 in]
      }
      frame "---------- Project ----------" {
        n118 = call <vilib>:"Add State(s) to Queue__jki_lib_state_machine.vi"("State(s) in (\"\")"=w317) -> ("States Out"=w316:string)  [unwired: 14 in]
      }
      frame "Project: Run Unit Tests" {
        # "Tests pass"
        n119 = Unbundle By Name(w338) -> ("RunningAsCmdLine"=w337:bool, "Build.Unit Test"=w327:path)
        n120 = property on="Tests Pass" class="Bool (strict)"(error in=w329, "Value"=FALSE ("Unit Tests Pass")) -> (error out=w326:errorcluster)  [unwired: 1 in, 1 out]
        n121 = call <userlib>:"Current VIs Parent Directory__ogtk.vi"("Relative path (.)"=path "Support VIs/Run Project Unit Tests Dynamically.vi" ("VI Path")) -> ("Parent Directory (+ Relative)"=w322:path)  [unwired: 4 in]
        n122 = Open VI Reference(type specifier VI Refnum (for type only)=refnum<vi> refnum, vi path=w322, error in (no error)=w326) -> (vi reference=w333:refnum<vi>, error out=w332:errorcluster)  [unwired: 3 in]
        n123 = call-by-ref "?"(reference=w333, error in=w332, "error in"=w332, "TestSuite"=w327) -> (reference out=w331:refnum<vi>, error out=w330:errorcluster, 0:"error out"=w325:errorcluster, "test details"=w319:string, "successful?"=w320:bool)  [unwired: 7 in]
        "Tests Pass" <- w320
        "Unit Test Results" <- w319
        n124 = Close Reference(reference=w331, error in (no error)=w330) -> (error out=w323:errorcluster)
        n125 = case "Abort Build (Test Failure)" shown="True" w320 {
          tunnel: w337 -> [w344 _]
          tunnel: [w349 w351] -> w335
          tunnel: w336 -> [_ w351]
          tunnel: w319 -> [w347 _]
          tunnel: [w341 _] -> w318
          frame False {
            w340 = 42 items=["No error", "Argument error", "Memory is full", "Out of zone", "End of file", "File already open", "Generic file I/O error", "File not found", "File permission error", "Disk is full", "Duplicate path", "Too many files open", "System feature not enabled", "Resource file not found", "Cannot add resource", "Resource not found", "Image not found", "Image memory error", "Pen does not exist", "Config type invalid", "Config token not found", "Config parse error", "Config memory error", "Bad external code format", "Bad external code offset", "External code not present", "Null window", "Destroy window error", "Null menu", "Print aborted", "Bad print record", "Print driver error", "Windows error during printing", "Memory error during printing", "Print dialog error", "Generic print error", "Invalid device refnum", "Device not found", "Device parameter error", "Device unit error", "Cannot open device", "Device call aborted", "Generic error", "Cancelled by user", "Object ID too low", "Object ID too high", "Object not in heap", "Unknown heap", "Unknown object (invalid DefProc)", "Unknown object (DefProc not in table)", "Message out of range", "Invalid (null) method", "Unknown message", "Manager call not supported", "Bad address", "Network operation in progress", "Network operation timed out", "Connection is busy", "Network attribute not supported", "Network error", "Address in use", "System out of memory", "Connection aborted", "Connection refused", "Not connected", "Already connected", "Connection closed", "Initialization error (interapplication manager)", "Bad occurrence", "Wait on unbound occurrence handler", "Occurrence queue overflow", "Datalog type conflict", "Unused", "Unrecognized type (interapplication manager)", "Memory corrupt", "Failed to make temporary DLL", "Old CIN version", "Drag socket not found", "Failed to load drop-object", "Failed to register OLE object", "Failed to release OLE object", "Format specifier type mismatch", "Unknown format specifier", "Too few format specifiers", "Too many format specifiers", "Scan failed", "Newer CIN version", "Error converting to variant", "Runtime menu error", "Password tampered", "Variant attribute not found", "Incompatible variant data type", "Event data is not available", "Event Store is not present", "Occurrence is not found", "Event Queue is not created", "Event info is not available", "Refnum passed is NULL", "Error retrieving Class GUID", "Error retrieving CoClass GUID", "Error retrieving TypeLib GUID.", "Bad built application magic bytes.", "Specific driver is different from the specific driver associated with the Logical Name.", "There is no session opened to the class driver.", "Max Error", "MAX - Error with config objects", "MAX - Error loading configuration", "MAX - Group not supported"]
            n126 = Format Into String(format string="Unit test failures: %s", w347) -> (resulting string=w345:string)  [unwired: 2 in, 1 out]
            n127 = call <vilib>:"Error Cluster From Error Code.vi"("error message (\"\")"=w345, "error code (0)"=w340) -> ("error out"=w343:errorcluster)  [unwired: 7 in]
            n128 = Select(t=w343, s=w344, f=errorcluster {"status"=FALSE, "code"=0, "source"=""}) -> (s? t:f=w341:errorcluster)
            n129 = Select(t="Macro: Exit" ("Text.Text"), s=w344, f="UI: Update Progress Status >> Aborted: Unit Test Failure\nMacro: End Build" ("Text.Text")) -> (s? t:f=w349:string)
          }
          frame True {
          }
        }
        n130 = call <vilib>:"Add State(s) to Queue__jki_lib_state_machine.vi"("State(s) in (\"\")"=w335) -> ("States Out"=w339:string)  [unwired: 14 in]
        n131 = Merge Errors(w323, w325, w318) -> (w324:errorcluster)
      }
      frame "Project: Copy .config" {
        n132 = property class="App"(error in=w356) -> (error out=w353:errorcluster, "App.VersionYear"=w355:string)  [unwired: 1 in, 1 out]
        n133 = Unbundle By Name(w357) -> ("CmdLineArgs.Workspace"=w352:path)
        n134 = case shown="Default" w355 {
          tunnel: [w361 w363] -> w354
          tunnel: w353 -> [w362 w363]
          tunnel: w352 -> [w360 _]
          frame Default {
            n135 = call "Copy Config to All Projects.vi"("error in (no error)"=w362, "Workspace dir"=w360) -> ("error out"=w361:errorcluster)  [unwired: 9 in]
          }
          frame "2010" {
          }
        }
        n136 = call <vilib>:"Add State(s) to Queue__jki_lib_state_machine.vi"("State(s) in (\"\")"=w359) -> ("States Out"=w358:string)  [unwired: 14 in]
      }
      frame "Project: Build" {
        # "2010 doesn't have public app builder api so make dynamic call to file location based upon version. they have same con pane\n2012 changed the 2011 to a polymorphic VI"
        n137 = Unbundle By Name(w380) -> ("CmdLineArgs"=w364:T3, "Build.Builds"=w369:T6[], "CmdLineArgs.SourceVer"=w368:string, "CmdLineArgs.BuildNumber"=w365:u32)
        n138 = property class="App"(error in=w379) -> (error out=w377:errorcluster, "App.VersionYear"=w366:string)  [unwired: 1 in, 1 out]
        n139 = VI Library() -> (path=w371:path)
        n140 = case shown="Default" w366 {
          tunnel: w371 -> [w385 w388 w391]
          tunnel: [w383 w386 w389] -> w370
          frame "2010" {
            n141 = Build Path(base path=w385, name or relative path="AppBuilder\\BuildTargetBuildSpecification.vi") -> (appended path=w383:path)
          }
          frame "2011" {
            n142 = Build Path(base path=w388, name or relative path="AppBuilder\\AB_API_Simple\\Build.vi") -> (appended path=w386:path)
          }
          frame Default {
            n143 = Build Path(base path=w391, name or relative path="AppBuilder\\AB_API_Simple\\Build (path).vi") -> (appended path=w389:path)
          }
        }
        n144 = Not Equal?(x=w368, y=w366) -> (x != y?=w367:bool)
        n145 = Open VI Reference(type specifier VI Refnum (for type only)=refnum<vi> refnum, vi path=w370, error in (no error)=w377) -> (vi reference=w376:refnum<vi>, error out=w378:errorcluster)  [unwired: 3 in]
        n146 = for {
          shift-right: [w396] -> w374
          shift-left: w378 -> [w397]
          tunnel: w369 -> [w399] mode=indexing
          shift-right: [w395] -> w373
          shift-left: w376 -> [w398]
          tunnel: w367 -> [w394]
          tunnel: w365 -> [w393]
          tunnel: w364 -> [w392]
          n147 = call "Build Action.vi"("Build number"=w393, "CmdLineArgs"=w392, "error in"=w397, "VerMismatch?"=w394, "Build Spec Info"=w399, "App Builder VI in"=w398) -> ("error out"=w396:errorcluster, "App Builder VI out"=w395:refnum<vi>)  [unwired: 4 in]
        }
        n148 = Close Reference(reference=w373, error in (no error)=w374) -> (error out=w372:errorcluster)
        n149 = call <vilib>:"Add State(s) to Queue__jki_lib_state_machine.vi"("State(s) in (\"\")"=w382) -> ("States Out"=w381:string)  [unwired: 14 in]
      }
      frame "Clear Compiled Obj Cache" {
        n150 = property class="App"(error in=w403) -> (error out=w400:errorcluster, "App.VersionYear"=w402:string)  [unwired: 1 in, 1 out]
        n151 = case shown="\"2010\"" w402 {
          tunnel: [w407 w409] -> w401
          tunnel: w400 -> [w408 w409]
          frame "2010" {
            # "2010 has all sorts of errors building the AIT 429 custom device without this set"
            n152 = invoke class="App" method="ClearCompObjCache"(error in=w408) -> (error out=w407:errorcluster)  [unwired: 2 in, 2 out]
          }
          frame Default {
          }
        }
        n153 = call <vilib>:"Add State(s) to Queue__jki_lib_state_machine.vi"("State(s) in (\"\")"=w406) -> ("States Out"=w405:string)  [unwired: 14 in]
      }
      frame "Project: Copy to Built" {
        n154 = Unbundle By Name(w419) -> ("Build.Retain Build"=w410:bool, "CmdLineArgs.Copy Built"=w411:bool, "RunningAsCmdLine"=w418:bool, "CmdLineArgs.BuildNumber"=w417:u32, "CmdLineArgs.Job"=w414:string, "CmdLineArgs.Workspace"=w415:path)
        n155 = And(x=w411, y=w418) -> (x .and. y?=w412:bool)
        n156 = case shown="True" w412 {
          tunnel: w417 -> [_ w427]
          tunnel: w416 -> [w422 w428]
          tunnel: w415 -> [_ w425]
          tunnel: w414 -> [_ w426]
          tunnel: [w422 w424] -> w413
          tunnel: w410 -> [_ w423]
          frame False {
          }
          frame True {
            n157 = call "Copy Build to Shared Location.vi"("Retain Build"=w423, "error in (no error)"=w428, "Workspace"=w425, "Job"=w426, "Build Number"=w427) -> ("error out"=w424:errorcluster)  [unwired: 6 in]
          }
        }
        n158 = call <vilib>:"Add State(s) to Queue__jki_lib_state_machine.vi"("State(s) in (\"\")"=w421) -> ("States Out"=w420:string)  [unwired: 14 in]
      }
    }
  }
  n159 = disable-structure shown="Enabled" {
    disable-tunnel: w2 -> [w429 _]
    frame Disabled {
      n160 = Close File(refnum=w429) -> ()  [unwired: 1 in, 2 out]
    }
    frame Enabled {
    }
  }
  n161 = Quit LabVIEW(quit? (T)=w1) -> ()
